vi "0036-Sub_-55C.vi"(11 "数値入力":dbl) -> (3 "数値出力":dbl)   [LabVIEW 2014]
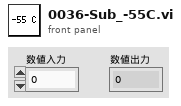
[diagram p1: front panel]
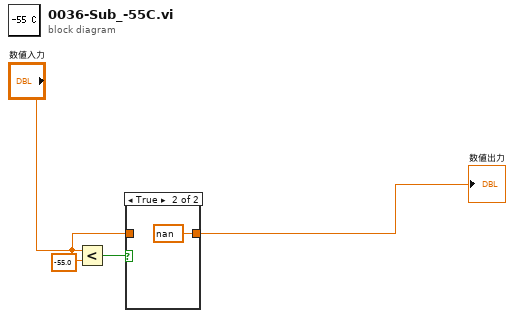
[diagram p0: block diagram]
diagram:
  n1 = Less?(x="数値入力", y=-55.0) -> (x < y?=w1:bool)
  n2 = case shown="TRUE" w1 {
    tunnel: [w5 nan ("数値")] -> w4
    tunnel: "数値入力" -> [w5 _]
    frame False {
    }
    frame True {
    }
  }
  "数値出力" <- w4
